vi "CMRR.vi"(11 "数组":dbl[](array[numeric])) -> (3 "KCMRR":dbl=118.45179628787717)   [LabVIEW 2019]
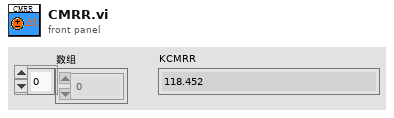
[diagram p1: front panel]
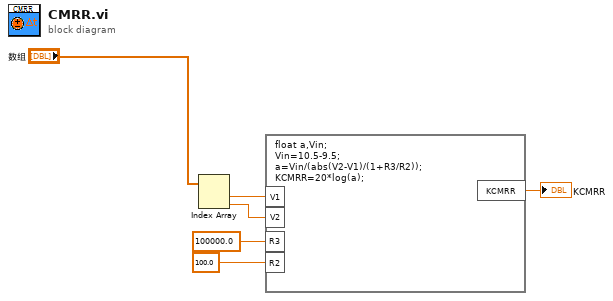
[diagram p0: block diagram]
diagram:
  n1 = Index Array(array="数组") -> (element #1=w1:dbl, element #2=w2:dbl)  [unwired: 2 in]
  n2 = formula code="float a,Vin;\nVin=10.5-9.5;\na=Vin/(abs(V2-V1)/(1+R3/R2));\nKCMRR=20*log(a);"("V1"=w1, "V2"=w2, "R3"=100000.0 ("输入变量"), "R2"=100.0 ("输入变量")) -> ("KCMRR"=→"KCMRR":dbl)
